vi "InitScope.vi"(10 "P2P params":T1={"instrument handle"="", "stream session"=refnum, "scale"={"offset"=0.0, "gain"=0.0, "reserved 1"=0.0, "reserved 2"=0.0}, "actual sample rate"=10000000.0, "Trigger"=enum."PFI 0"} {"actual sample rate" format="%.2p"}, 11 "FPGA VI Reference":T3) -> (3 "scope params":T4={"scope mode"=enum."Stopped", "ticker"=refnum, "record length"=0, "FPGA ref"=refnum, "P2P params"={"instrument handle"="", "stream session"=refnum, "scale"={"offset"=0.0, "gain"=0.0, "reserved 1"=0.0, "reserved 2"=0.0}, "actual sample rate"=10000000.0, "Trigger"=enum."PFI 0"}, "FPGA ref 5160"=refnum} {"P2P params"."actual sample rate" format="%.2p"})   [LabVIEW 2013]
uses:
  controls/scope_params.ctl
  Utilities/Ticker/Ticker.lvclass
  controls/ScopeMode.ctl
  Config/FPGAref.ctl
  P2P streaming/P2P params.ctl
  P2P streaming/trigger_source.ctl
  Config/5160FPGAref.ctl
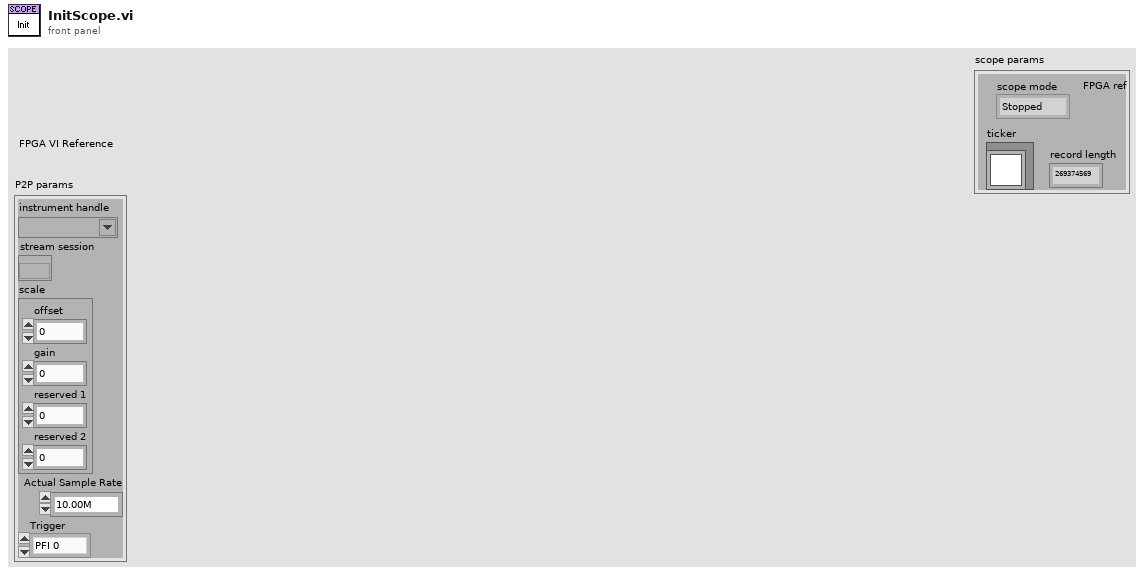
[diagram p1: front panel]
types:
  T1 = typedef "P2P params.ctl" = cluster{"instrument handle":refnum<k15>, "stream session":refnum<k20>, "scale":cluster{"offset":dbl, "gain":dbl, "reserved 1":dbl, "reserved 2":dbl}, "actual sample rate":dbl, "Trigger":T2}
  T2 = typedef "trigger_source.ctl" = enum16{"PFI 0", "PFI 1", "Software"}
  T3 = typedef "FPGAref.ctl" = refnum<k20>
  T4 = typedef "scope_params.ctl" = cluster{"scope mode":T5, "ticker":refnum<class "Ticker.lvclass">, "record length":u32, "FPGA ref":T3, "P2P params":T1, "FPGA ref 5160":T6}
  T5 = typedef "ScopeMode.ctl" = enum16{"Stopped", "Single", "Running"}
  T6 = typedef "5160FPGAref.ctl" = refnum<k20>
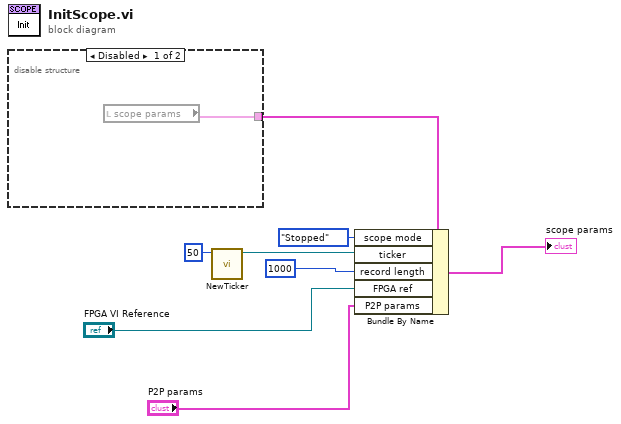
[diagram p0: block diagram]
diagram:
  n1 = disable-structure shown="Disabled" {
    disable-tunnel: [w9 _] -> w8
    frame Disabled {
      n2 = local read "scope params"() -> (w9:T4)
    }
    frame Enabled {
    }
  }
  n3 = call "NewTicker.vi"("Period"=u32 50) -> ("Ticker"=w5:refnum<class "Ticker.lvclass">)  [unwired: 10 in]
  n4 = Bundle By Name(cluster=w8, "scope mode"=ScopeMode."Stopped", "ticker"=w5, "record length"=u32 1000, "FPGA ref"="FPGA VI Reference", "P2P params"="P2P params") -> (→"scope params":T4)
